vi "Shared Variable GUID Lookup.vi"() -> ()   [LabVIEW 2015, in "Shared Variable Custom Device.lvlib"]
doc: "Use this Global VI to access the GUIDs assigned to the page resources of the Custom Device."
uses:
  Shared Variable Custom Device.lvlib
panel:
  in  "Error Code Page GUID":string="ddf28850-23ce-4531-82d8-c13825fbca57"
  in  "Connection Status Page GUID":string="78b8a558-7db9-4af3-b3a2-92998c4dbfe3"
  in  "Read Page GUID":string="56684d90-57c0-46bf-95c3-c3ec5ca5eaaf"
  in  "Write Page GUID":string="efcd8c5b-4fff-4983-a7df-34ee49fee23a"
  in  "Status Page GUID":string="1e09d8c3-69f5-401b-b7dc-c892426ca993"
  in  "Boolean Page GUID":string="40ef8b4b-fafe-4302-bf5b-f1049513b872"
  in  "String Page GUID":string="4a3273d2-25cf-4c75-aa6c-6d863714b97d"
  in  "Double Page GUID":string="745b2fb1-1cbc-4e0d-8c6b-85ee92b63937"
  in  "Custom Device Page GUID":string="f341660c-60a9-4d85-aa66-ad00d8329358"
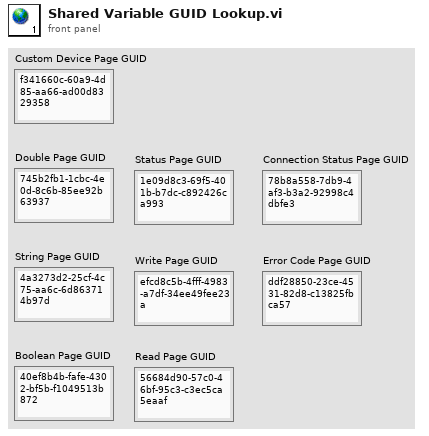
[diagram p1: front panel]
diagram:
